vi "support.path_to_string.vi"(11 "path":path) -> (3 "path as string":string)   [LabVIEW 2020, in "reqwest.lvlib"]
uses:
  RequestBuilder/RequestBuilder.lvclass/RequestBuilder.ctl
  reqwest.lvlib
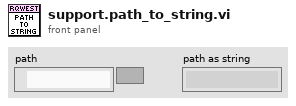
[diagram p1: front panel]
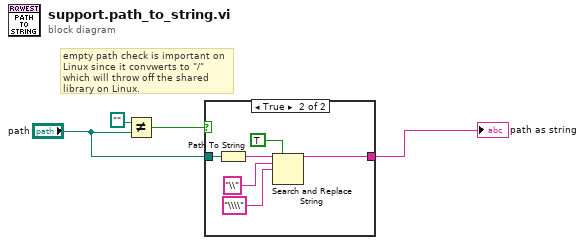
[diagram p0: block diagram]
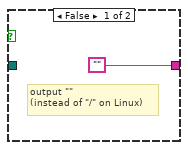
[diagram p2: hidden frame]
diagram:
  # "empty path check is important on Linux since it convwerts to \"/\" which will throw off the shared library on Linux."
  n1 = Not Equal?(x=path "", y="path") -> (x != y?=w1:bool)
  n2 = case shown="True" w1 {
    tunnel: "path" -> [_ w7]
    tunnel: ["" w6] -> w3
    frame False {
      # "output \"\"\n(instead of \"/\" on Linux)"
    }
    frame True {
      n3 = Path To String(path=w7) -> (string=w11:string)
      n4 = Search and Replace String(replace all?=TRUE ("replace all? (F)"), input string=w11, search string="\\", replace string="\\\\" ("replace string (\"\")")) -> (result string=w6:string)  [unwired: 4 in, 3 out]
    }
  }
  "path as string" <- w3
